vi "Signal Get Dimension.vi"(8 "error in (no error)":errorcluster, 11 "Signal DVR in":refnum<data-value>) -> (0 "error out":errorcluster, 2 "Dimension out":refnum<data-value>, 3 "Signal DVR out":refnum<data-value>)   [LabVIEW 2010, in "MDSplus.lvlib"]
uses:
  <vilib>/MDSplus/Library/MDSplus.lvlib
  <vilib>/MDSplus/Classes/Data_Class/Data.lvclass
  <vilib>/MDSplus/Classes/Data_Class/Compound_Class/Signal_Class/Signal.lvclass
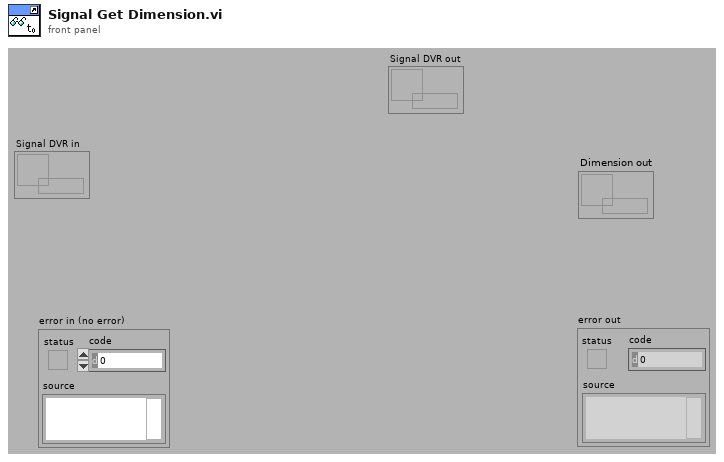
[diagram p1: front panel]
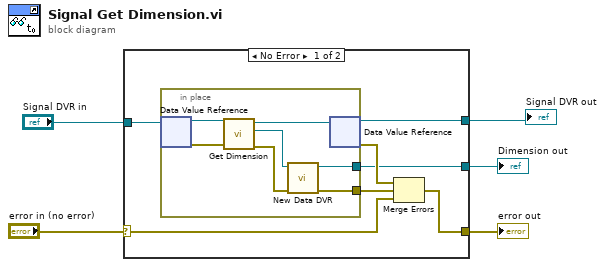
[diagram p0: block diagram]
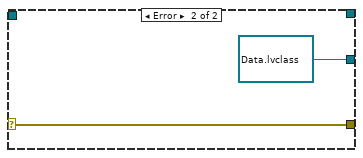
[diagram p2: hidden frame]
diagram:
  n1 = case shown="No Error" "error in (no error)" {
    selector: "error in (no error)" -> [w12 w21]
    tunnel: [w10 w21] -> w5
    tunnel: [w8 refnum<data-value> refnum ("Data DVR")] -> w3
    tunnel: "Signal DVR in" -> [w7 _]
    tunnel: [w6 _] -> w1
    frame No Error {
      n2 = in-place {
        in-place-border: [w19] -> w8
        in-place-border: [w18] -> w9
        n3 = in-place-dvr #1(w7) -> (w17:refnum<class "Signal.lvclass">, w16:errorcluster)
        n4 = call <vilib>:"Get Dimension.vi"("error in (no error)"=w16, "Signal in"=w17) -> ("error out"=w14:errorcluster, "Ending out"=w13:refnum<class "Data.lvclass">, "Signal out"=w15:refnum<class "Signal.lvclass">)  [unwired: 7 in]
        n5 = call <vilib>:"New Data DVR.vi"("error in (no error)"=w14, "Data in"=w13) -> ("error out"=w18:errorcluster, "Data DVR out"=w19:refnum<data-value>)  [unwired: 8 in]
        n6 = in-place-dvr #1(w15) -> (w6:refnum<data-value>, w11:errorcluster)
      }
      n7 = Merge Errors(w11, w9, w12) -> (w10:errorcluster)
    }
    frame Error {
    }
  }
  "error out" <- w5
  "Dimension out" <- w3
  "Signal DVR out" <- w1
